vi "Measurement Configuration.vi"   [LabVIEW 2015, in "Keysight U1252.lvlib"]
uses:
  <instrlib>/Keysight U1252/Keysight U1252.lvlib
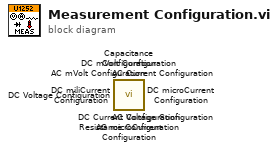
[diagram p0: block diagram]
diagram:
  n1 = call <instrlib>:"DC Current Configuration.vi"() -> ()  [unwired: 10 in, 2 out]
  n2 = call <instrlib>:"AC Current Configuration.vi"() -> ()  [unwired: 10 in, 2 out]
  n3 = call <instrlib>:"DC miliCurrent Configuration.vi"() -> ()  [unwired: 10 in, 2 out]
  n4 = call <instrlib>:"DC microCurrent Configuration.vi"() -> ()  [unwired: 10 in, 2 out]
  n5 = call <instrlib>:"AC microCurrent Configuration.vi"() -> ()  [unwired: 10 in, 2 out]
  n6 = call <instrlib>:"Capacitance Configuration.vi"() -> ()  [unwired: 10 in, 2 out]
  n7 = call <instrlib>:"AC mVolt Configuration.vi"() -> ()  [unwired: 10 in, 2 out]
  n8 = call <instrlib>:"DC mVolt Configuration.vi"() -> ()  [unwired: 10 in, 2 out]
  n9 = call <instrlib>:"DC Voltage Configuration.vi"() -> ()  [unwired: 10 in, 2 out]
  n10 = call <instrlib>:"Resistance Configuration.vi"() -> ()  [unwired: 10 in, 2 out]
  n11 = call <instrlib>:"AC Voltage Configuration.vi"() -> ()  [unwired: 10 in, 2 out]
